vi "Telescope Move Focus.vi"(8 "error in (no error)":errorcluster, 10 "Focus Pos":dbl, 11 "PRIME Telescope in":refnum<class "PRIME Telescope.lvclass">) -> (0 "error out":errorcluster, 3 "PRIME Telescope out":refnum<class "PRIME Telescope.lvclass">)   [LabVIEW 2021, in "PRIME Telescope.lvclass"]
uses:
  PRIME Telescope.lvclass
  PRIME Telescope.lvclass/PRIME Telescope.ctl
  Telescope.lvclass
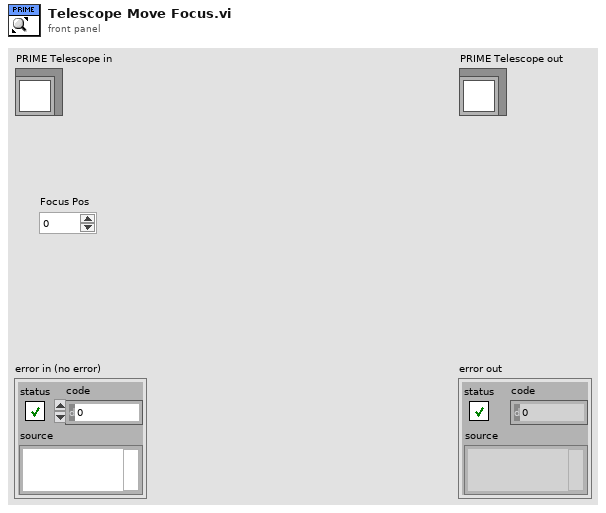
[diagram p1: front panel]
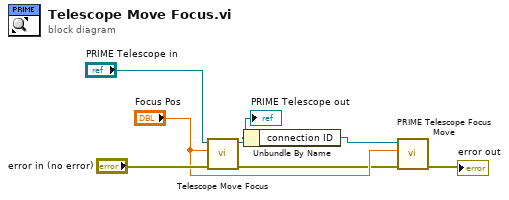
[diagram p0: block diagram]
diagram:
  n1 = call-parent "Telescope Move Focus.vi"("error in (no error)"="error in (no error)", "Focus Pos"="Focus Pos", "Telescope in"="PRIME Telescope in") -> ("error out"=w2:errorcluster, "Telescope out"=w5:refnum<class "PRIME Telescope.lvclass">)  [unwired: 7 in]
  "PRIME Telescope out" <- w5
  n2 = Unbundle By Name(w5) -> ("connection ID"=w4:refnum<k5>)
  n3 = call "PRIME Telescope Focus Move.vi"("error in (no error)"=w2, "focus pos"="Focus Pos", "connection ID"=w4) -> ("error out"=→"error out":errorcluster)  [unwired: 8 in]
